vi "DequeueMessage.vi"(8 "error in (no error)":errorcluster, 11 "queue in":T1) -> (0 "error out":errorcluster, 1 "Data (Variant)":variant, 2 "Message":string, 3 "queue out (copy)":T1)   [LabVIEW 2020]
uses:
  QueueRef.ctl
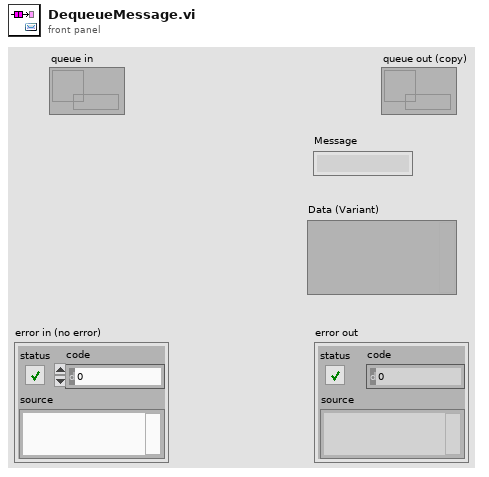
[diagram p1: front panel]
types:
  T1 = typedef "QueueRef.ctl" = refnum<queue>
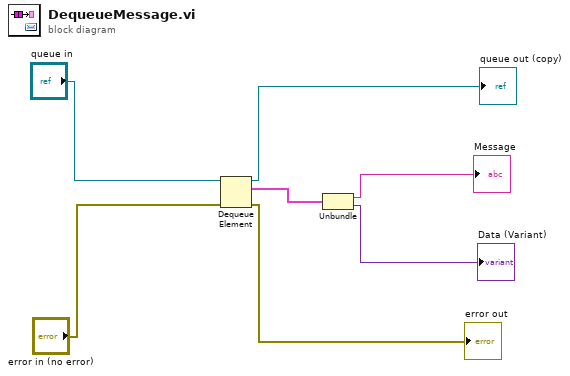
[diagram p0: block diagram]
diagram:
  n1 = Dequeue Element(queue="queue in", error in (no error)="error in (no error)") -> (queue out=→"queue out (copy)":T1, element=w3:cluster{string, "element data type":variant}, error out=→"error out":errorcluster)  [unwired: 1 in, 1 out]
  n2 = Unbundle(w3) -> (→"Message":string, "element data type"=→"Data (Variant)":variant)
